vi "FGV_Calibration_KeyParams.vi"(7 "Action":T5, 8 "error in (no error)":errorcluster, 10 "GFG varname (Query)":string, 11 "System Type":string) -> (0 "error out":errorcluster, 1 "Imaging Reso Key Parameters":T4, 2 "Imaging Galvo Key Parameters":T4, 3 "Stimulating Galvo Key Parameters":T4, 4 "GFG Value requested":variant, 5 "Error Status Array (Empty on no error)":T1[](array[typedef]))   [LabVIEW 2012]
uses:
  Custom Controls and Typedefs/FGV_CalibrationKeyParams_Actions.ctl
  Custom Controls and Typedefs/Calibration Key Param structure.ctl
  <vilib>/Utility/VariantDataType/Type.ctl
  GFG/GFG Translator Wrapper/GFGTranslator_errors.ctl
  Custom Controls and Typedefs/Galvo Key Parameters.ctl
  Custom Controls and Typedefs/Reso Key Parameters.ctl
  Custom Controls and Typedefs/Galvo (Stim Path) Key Parameters.ctl
  GFG/GFG Translator Wrapper/GFGTranslator_Action.ctl
  GFG/GFG Translator Wrapper/GFGTranslator_Datatype.ctl
  Global_CalibrationSimulation.vi
  <vilib>/Utility/config.llb/Read Key (Double).vi
  <vilib>/Utility/config.llb/Read Key (Boolean).vi
  <vilib>/Utility/config.llb/NI_LVConfig.lvlib
  <vilib>/Utility/VariantDataType/VariantType.lvlib
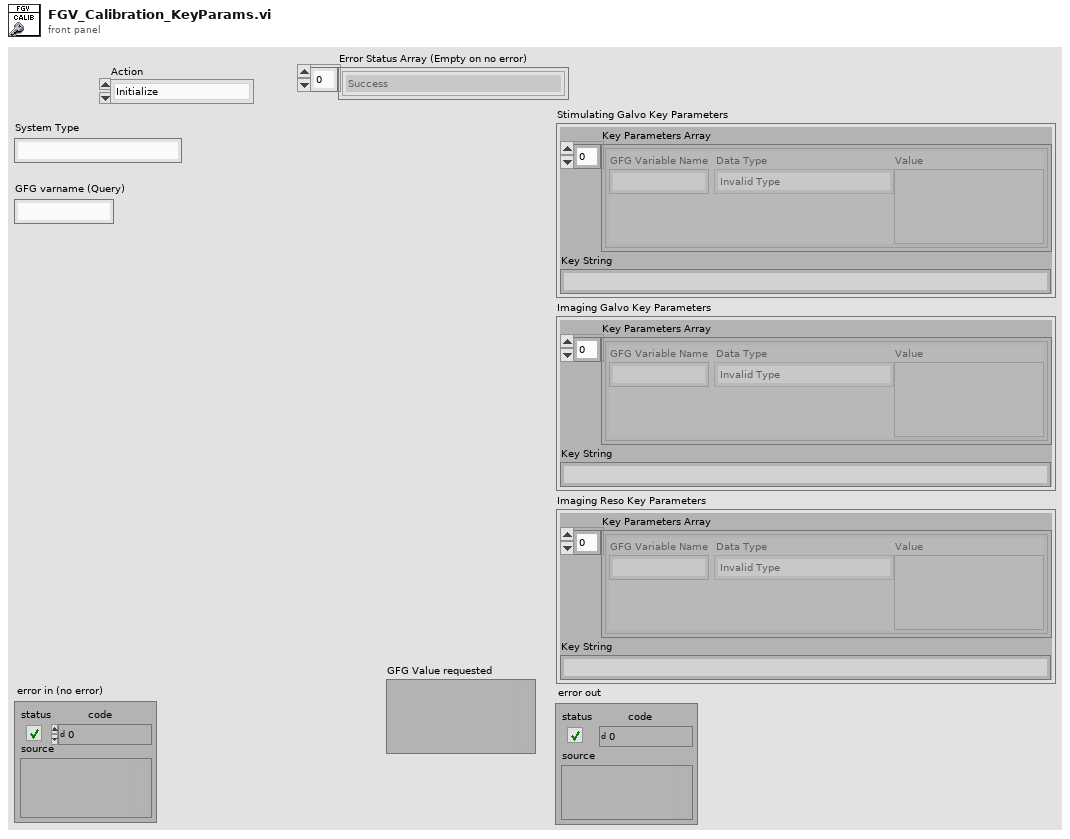
[diagram p1: front panel]
types:
  T1 = typedef "GFGTranslator_errors.ctl" = enum16{"Success", "SciScan Not Running", "No Get Method for Selected Datatype", "No Set Method for Selected Datatype", "Variable Not Found", "Unexpected Datatype", "Data Out of Range"}
  T2 = typedef "Calibration Key Param structure.ctl" = cluster{"GFG Variable Name":string, "Data Type":T3, "Value":variant}
  T3 = typedef "VariantType.lvlib/Type.ctl" = enum8{"Invalid Type", "Void", "I8", "I16", "I32", "I64", "U8", "U16", "U32", "U64", "Single Float", "Double Float", "Extended Float", "Single Complex", "Double Complex", "Extended Complex", "Enum U8", "Enum U16", "Enum U32", "Enum U64", "Single Float With Unit", "Double Float With Unit", "Extended Float With Unit", "Single Complex with Unit", "Double Complex with Unit", "Extended Complex with Unit", "Boolean", "String", "Path", "Picture", "Tag", "Array", "Cluster", "Variant", "LV Variant", "Waveform", "Timestamp", "Digital Waveform", "Digital Data", "ExpressData", "Refnum", "External Data", "VI", "Poly VI", "LabVIEW Class Instance", "Fixed Point"}
  T4 = cluster{"Key Parameters Array":T2[], "Key String":string}
  T5 = typedef "FGV_CalibrationKeyParams_Actions.ctl" = enum16{"Initialize", "Grab From SciScan and Store", "Read Parameters", "ReadGFGValue"}
  T6 = typedef "Galvo (Stim Path) Key Parameters.ctl" = T2[]
  T7 = typedef "Reso Key Parameters.ctl" = T2[]
  T8 = typedef "Galvo Key Parameters.ctl" = T2[]
  T9 = typedef "GFGTranslator_Datatype.ctl" = enum16{"String", "Path (String)", "Numeric", "Boolean", "Set_BoolRef (use boolean data)", "Get_Variant", "Get_2DArray (I16)", "Get_Image_2DArray (I16)", "Get_Version (String)", "Get_All GFG variables (String)"}
  T10 = typedef "GFGTranslator_Action.ctl" = enum16{"Get", "Set"}
  T11 = typedef "NI_LVConfig.lvlib/Config Data RefNum.ctl" = refnum<k1>
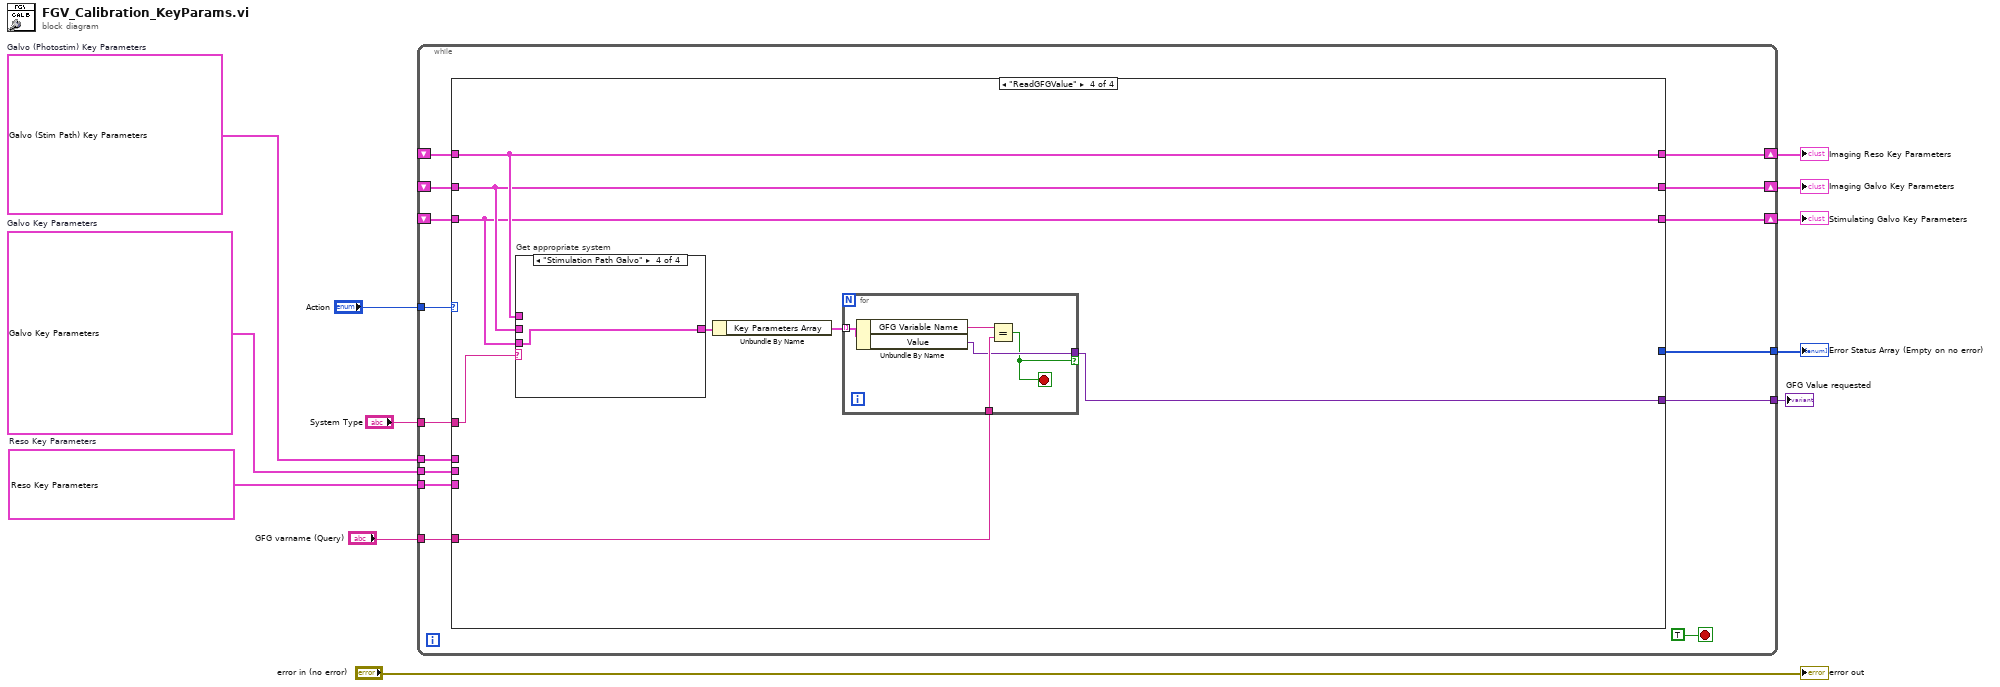
[diagram p0: block diagram]
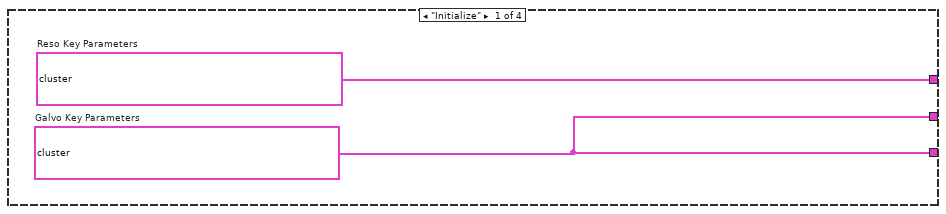
[diagram p2: hidden frame]
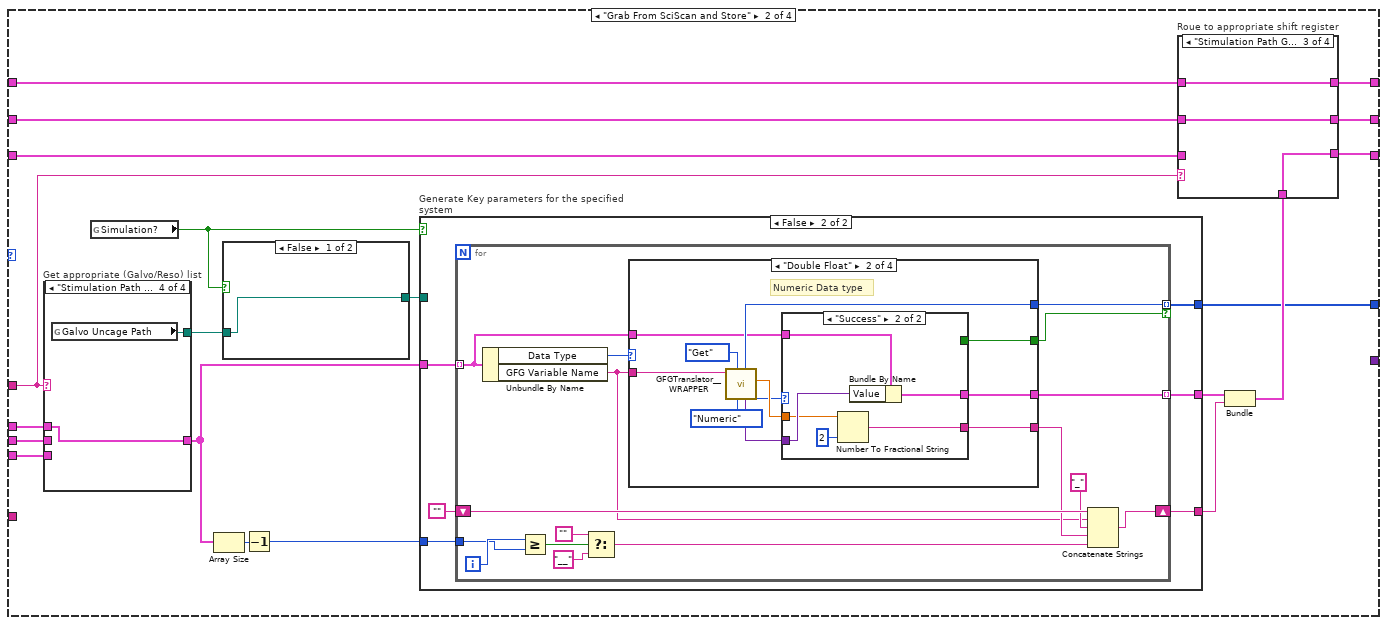
[diagram p3: hidden frame]
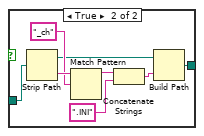
[diagram p4: hidden frame]
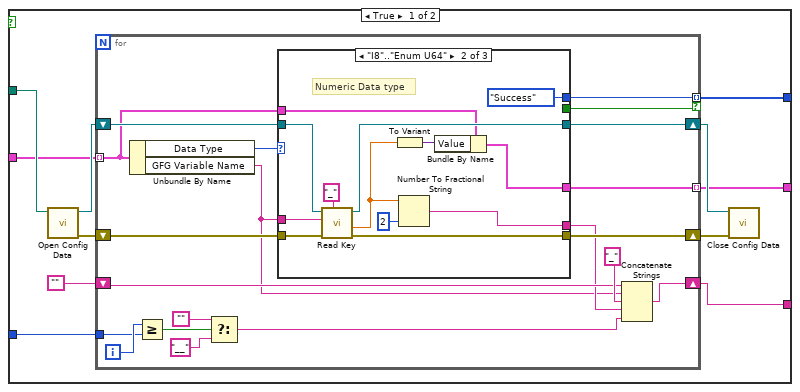
[diagram p5: hidden frame]
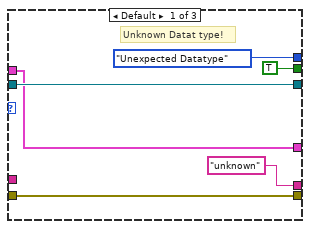
[diagram p6: hidden frame]
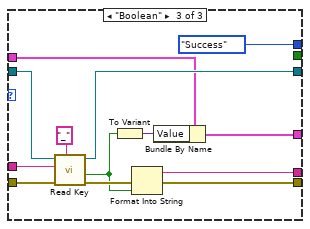
[diagram p7: hidden frame]
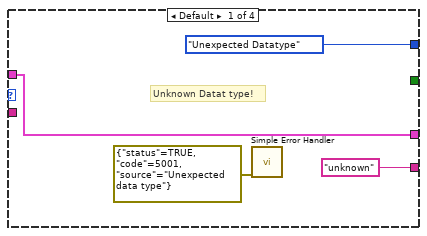
[diagram p8: hidden frame]
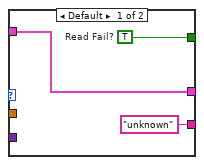
[diagram p9: hidden frame]
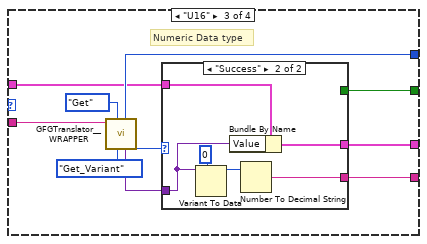
[diagram p10: hidden frame]
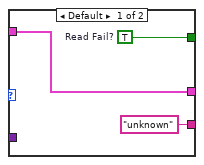
[diagram p11: hidden frame]
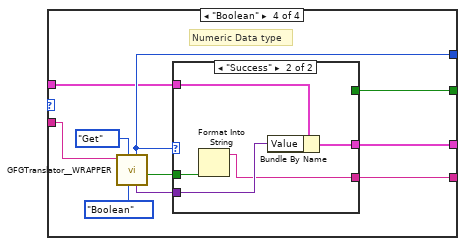
[diagram p12: hidden frame]
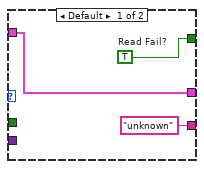
[diagram p13: hidden frame]
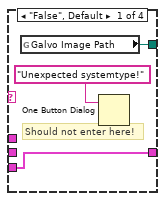
[diagram p14: hidden frame]
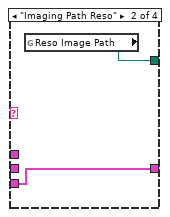
[diagram p15: hidden frame]
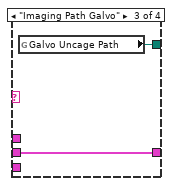
[diagram p16: hidden frame]
diagram:
  w3 = T6 [{"GFG Variable Name"="x.voltage", "Data Type"=enum."Double Float", "Value"=variant}, {"GFG Variable Name"="y.voltage", "Data Type"=enum."Double Float", "Value"=variant}, {"GFG Variable Name"="x.volt.offset", "Data Type"=enum."Double Float", "Value"=variant}, {"GFG Variable Name"="y.volt.offset", "Data Type"=enum."Double Float", "Value"=variant}, {"GFG Variable Name"="fill.fraction", "Data Type"=enum."Double Float", "Value"=variant}, {"GFG Variable Name"="x.invert.image", "Data Type"=enum."Boolean", "Value"=variant}, {"GFG Variable Name"="y.invert.image", "Data Type"=enum."Boolean", "Value"=variant}]  # Galvo (Photostim) Key Parameters
  w8 = T7 [{"GFG Variable Name"="x.voltage", "Data Type"=enum."Double Float", "Value"=variant}, {"GFG Variable Name"="y.voltage", "Data Type"=enum."Double Float", "Value"=variant}, {"GFG Variable Name"="x.correction", "Data Type"=enum."Double Float", "Value"=variant}]  # Reso Key Parameters
  w9 = T8 [{"GFG Variable Name"="x.voltage", "Data Type"=enum."Double Float", "Value"=variant}, {"GFG Variable Name"="y.voltage", "Data Type"=enum."Double Float", "Value"=variant}, {"GFG Variable Name"="x.volt.offset", "Data Type"=enum."Double Float", "Value"=variant}, {"GFG Variable Name"="y.volt.offset", "Data Type"=enum."Double Float", "Value"=variant}, {"GFG Variable Name"="speed.mode", "Data Type"=enum."U16", "Value"=variant}, {"GFG Variable Name"="fill.fraction", "Data Type"=enum."Double Float", "Value"=variant}, {"GFG Variable Name"="x.bidirectional", "Data Type"=enum."Boolean", "Value"=variant}, {"GFG Variable Name"="y.bidirectional", "Data Type"=enum."Boolean", "Value"=variant}, {"GFG Variable Name"="x.invert.image", "Data Type"=enum."Boolean", "Value"=variant}, {"GFG Variable Name"="y.invert.image", "Data Type"=enum."Boolean", "Value"=variant}]  # Galvo Key Parameters
  n1 = while {
    tunnel: "Action" -> [w26]
    tunnel: "System Type" -> [w22]
    shift-right: [w23] -> w5
    shift-left: _ -> [w21]
    shift-right: [w24] -> w6
    shift-left: _ -> [w20]
    shift-right: [w25] -> w7
    shift-left: _ -> [w19]
    tunnel: w9 -> [w18]
    tunnel: w8 -> [w17]
    tunnel: [w16] -> w4
    tunnel: w3 -> [w15]
    tunnel: "GFG varname (Query)" -> [w14]
    tunnel: [w13] -> w1
    stop <- TRUE stop-if-true
    n2 = case shown="\"ReadGFGValue\"" w26 {
      tunnel: [w28 w36 w224 w232] -> w25
      tunnel: [w28 w40 w225 w233] -> w24
      tunnel: [w29 w35 w226 w234] -> w23
      tunnel: w22 -> [_ w46 _ w231]
      tunnel: w21 -> [_ w49 w226 w234]
      tunnel: w20 -> [_ w48 w225 w233]
      tunnel: w19 -> [_ w47 w224 w232]
      tunnel: w18 -> [_ w43 _ _]
      tunnel: w17 -> [_ w42 _ _]
      tunnel: [_ w34 _ _] -> w16
      tunnel: w15 -> [_ w30 _ _]
      tunnel: w14 -> [_ _ _ w228]
      tunnel: [_ _ _ w227] -> w13
      frame "Initialize" {
        w29 = T4 {"Key Parameters Array"=[{"GFG Variable Name"="x.voltage", "Data Type"=enum."Double Float", "Value"=variant}, {"GFG Variable Name"="y.voltage", "Data Type"=enum."Double Float", "Value"=variant}, {"GFG Variable Name"="x.correction", "Data Type"=enum."Double Float", "Value"=variant}, {"GFG Variable Name"="Start.Delay", "Data Type"=enum."Double Float", "Value"=variant}], "Key String"="__"}  # Reso Key Parameters
        w28 = T4 {"Key Parameters Array"=[{"GFG Variable Name"="x.voltage", "Data Type"=enum."Double Float", "Value"=variant}, {"GFG Variable Name"="y.voltage", "Data Type"=enum."Double Float", "Value"=variant}, {"GFG Variable Name"="x.volt.offset", "Data Type"=enum."Double Float", "Value"=variant}, {"GFG Variable Name"="y.volt.offset", "Data Type"=enum."Double Float", "Value"=variant}, {"GFG Variable Name"="Start.Delay", "Data Type"=enum."Double Float", "Value"=variant}, {"GFG Variable Name"="speed.mode", "Data Type"=enum."U16", "Value"=variant}, {"GFG Variable Name"="fill.fraction", "Data Type"=enum."Double Float", "Value"=variant}, {"GFG Variable Name"="x.bidirectional", "Data Type"=enum."Boolean", "Value"=variant}, {"GFG Variable Name"="y.bidirectional", "Data Type"=enum."Boolean", "Value"=variant}], "Key String"="__"}  # Galvo Key Parameters
      }
      frame "Grab From SciScan and Store" {
        n3 = case "Get appropriate (Galvo/Reso) list" shown="\"Stimulation Path Galvo\"" w46 {
          tunnel: w43 -> [_ _ w209 _]
          tunnel: w42 -> [w204 w207 _ _]
          tunnel: [w204 w207 w209 w210] -> w41
          tunnel: [w203 w206 w208 w211] -> w32
          tunnel: w30 -> [_ _ _ w210]
          frame "False", Default {
            # "Should not enter here!"
            n4 = global read "Global_CalibrationSimulation.vi" "Galvo Image Path"() -> (w203:path)
            n5 = One Button Dialog(message="Unexpected systemtype!") -> ()  [unwired: 1 in, 1 out]
          }
          frame "Imaging Path Reso" {
            n6 = global read "Global_CalibrationSimulation.vi" "Reso Image Path"() -> (w206:path)
          }
          frame "Imaging Path Galvo" {
            n7 = global read "Global_CalibrationSimulation.vi" "Galvo Uncage Path"() -> (w208:path)
          }
          frame "Stimulation Path Galvo" {
            n8 = global read "Global_CalibrationSimulation.vi" "Galvo Uncage Path"() -> (w211:path)
          }
        }
        n9 = global read "Global_CalibrationSimulation.vi" "Simulation?"() -> (w33:bool)
        n10 = Array Size(array=w41) -> (size(s)=w45:i32)
        n11 = case shown="False" w33 {
          tunnel: w32 -> [w50 w52]
          tunnel: [w50 w51] -> w31
          frame False {
          }
          frame True {
            n12 = Strip Path(path=w52) -> (stripped path=w54:path, name=w57:string)
            n13 = Match Pattern(string=w57, regular expression="_ch" ("search string")) -> (before substring=w55:string)  [unwired: 1 in, 3 out]
            n14 = Concatenate Strings(w55, ".INI" ("string")) -> (w53:string)
            n15 = Build Path(base path=w54, name or relative path=w53) -> (appended path=w51:path)
          }
        }
        n16 = Decrement(x=w45) -> (x-1=w44:i32)
        n17 = case "Generate Key parameters for the specified system" shown="False" w33 {
          tunnel: w31 -> [w69 _]
          tunnel: [w64 w127] -> w34
          tunnel: [w59 w126] -> w39
          tunnel: w44 -> [w62 w124]
          tunnel: [w60 w123] -> w38
          tunnel: w41 -> [w63 w122]
          frame True {
            n18 = call <vilib>:"Open Config Data.vi"("configuration file path"=w69) -> ("error out"=w67:errorcluster, "refnum"=w68:T11)  [unwired: 8 in, 1 out]
            n19 = for {
              shift-right: [w88] -> w65
              shift-left: w68 -> [w89]
              shift-right: [w86] -> w66
              shift-left: w67 -> [w87]
              tunnel: [w85] -> w64 mode=indexing if=w84
              tunnel: w63 -> [w73] mode=indexing
              tunnel: w62 -> [w80]
              shift-right: [w74] -> w60
              shift-left: "" -> [w78]
              tunnel: [w72] -> w59 mode=indexing
              i -> [w81]
              n20 = Unbundle By Name(w73) -> ("Data Type"=w83:T3, "GFG Variable Name"=w76:string)
              n21 = Greater Or Equal?(x=w81, y=w80) -> (x >= y?=w82:bool)
              n22 = Select(t="", s=w82, f="__" ("t")) -> (s? t:f=w75:string)
              n23 = case shown="\"I8\"..\"Enum U64\"" w83 {
                tunnel: w76 -> [_ w102 w116]
                tunnel: w89 -> [w94 w107 w120]
                tunnel: [w94 w106 w119] -> w88
                tunnel: w87 -> [w95 w105 w118]
                tunnel: [w95 w103 w113] -> w86
                tunnel: [GFGTranslator_errors."Unexpected Datatype" ("Status Output") GFGTranslator_errors."Success" ("Status Output") GFGTranslator_errors."Success" ("Status Output")] -> w85
                tunnel: [TRUE _ _] -> w84
                tunnel: ["unknown" w100 w114] -> w77
                tunnel: w73 -> [w91 w99 w112]
                tunnel: [w91 w96 w109] -> w72
                frame Default {
                  # "Unknown Datat type!"
                }
                frame "I8".."Enum U64" {
                  # "Numeric Data type"
                  n24 = call-poly <vilib>:"Read Key.vi"("section"="_", "error in (no error)"=w105, "key"=w102, "refnum"=w107) -> ("error out"=w103:errorcluster, "value"=w97:dbl, "refnum out"=w106:T11)  [unwired: 4 in, 1 out]
                  n25 = To Variant(anything=w97) -> (Variant=w98:variant)
                  n26 = Number To Fractional String(number=w97, precision (6)=i16 2) -> (F-format string=w100:string)  [unwired: 2 in]
                  n27 = Bundle By Name(cluster=w99, "Value"=w98) -> (w96:T2)
                }
                frame "Boolean" {
                  n28 = call-poly <vilib>:"Read Key.vi"("section"="_", "error in (no error)"=w118, "key"=w116, "refnum"=w120) -> ("error out"=w115:errorcluster, "value"=w111:bool, "refnum out"=w119:T11)  [unwired: 4 in, 1 out]
                  n29 = To Variant(anything=w111) -> (Variant=w110:variant)
                  n30 = Format Into String(error in=w115, w111) -> (resulting string=w114:string, error out=w113:errorcluster)  [unwired: 2 in]
                  n31 = Bundle By Name(cluster=w112, "Value"=w110) -> (w109:T2)
                }
              }
              n32 = Concatenate Strings(w78, w76, "_" ("string"), w77, w75) -> (w74:string)
            }
            n33 = call <vilib>:"Close Config Data.vi"("error in (no error)"=w66, "refnum"=w65) -> ()  [unwired: 8 in, 2 out]
          }
          frame False {
            n34 = for {
              tunnel: [w143] -> w127 mode=indexing if=w142
              tunnel: [w141] -> w126 mode=indexing
              shift-right: [w134] -> w123
              shift-left: "" -> [w140]
              tunnel: w124 -> [w137]
              tunnel: w122 -> [w132] mode=indexing
              i -> [w138]
              n35 = Unbundle By Name(w132) -> ("Data Type"=w133:T3, "GFG Variable Name"=w130:string)
              n36 = Greater Or Equal?(x=w138, y=w137) -> (x >= y?=w136:bool)
              n37 = Select(t="", s=w136, f="__" ("t")) -> (s? t:f=w135:string)
              n38 = case shown="\"Double Float\"" w133 {
                tunnel: w130 -> [_ w148 w167 w185]
                tunnel: [GFGTranslator_errors."Unexpected Datatype" ("Status Output") w154 w173 w192] -> w143
                tunnel: [_ w153 w172 w191] -> w142
                tunnel: [w144 w151 w170 w187] -> w141
                tunnel: ["unknown" w150 w169 w186] -> w139
                tunnel: w132 -> [w144 w149 w168 w189]
                frame Default {
                  # "Unknown Datat type!"
                  n39 = call <vilib>:"Simple Error Handler.vi"("error in (no error)"=errorcluster {"status"=TRUE, "code"=5001, "source"="Unexpected data type"} ("error constant")) -> ()  [unwired: 4 in, 5 out]
                }
                frame "Double Float" {
                  # "Numeric Data type"
                  n40 = call "GFGTranslator__WRAPPER.vi"("GFGTranslator Datatype"=GFGTranslator_Datatype."Numeric", "GFG Translator Action"=GFGTranslator_Action."Get", "GFG Variable Name"=w148) -> ("Numeric_Output"=w155:dbl, "Variant_Output"=w152:variant, "Status Output"=w154:T1)  [unwired: 3 in, 3 out]
                  n41 = case shown="\"Success\"" w154 {
                    tunnel: w155 -> [_ w164]
                    tunnel: [w160 _] -> w153
                    tunnel: w152 -> [_ w166]
                    tunnel: [w159 w165] -> w151
                    tunnel: ["unknown" w162] -> w150
                    tunnel: w149 -> [w159 w161]
                    frame Default {
                      w160 = TRUE  # Read Fail?
                    }
                    frame "Success" {
                      n42 = Number To Fractional String(number=w164, precision (6)=i16 2) -> (F-format string=w162:string)  [unwired: 2 in]
                      n43 = Bundle By Name(cluster=w161, "Value"=w166) -> (w165:T2)
                    }
                  }
                }
                frame "U16" {
                  # "Numeric Data type"
                  n44 = call "GFGTranslator__WRAPPER.vi"("GFGTranslator Datatype"=GFGTranslator_Datatype."Get_Variant", "GFG Translator Action"=GFGTranslator_Action."Get", "GFG Variable Name"=w167) -> ("Variant_Output"=w171:variant, "Status Output"=w173:T1)  [unwired: 3 in, 4 out]
                  n45 = case shown="\"Success\"" w173 {
                    tunnel: [w178 _] -> w172
                    tunnel: w171 -> [_ w181]
                    tunnel: [w177 w184] -> w170
                    tunnel: ["unknown" w183] -> w169
                    tunnel: w168 -> [w177 w182]
                    frame Default {
                      w178 = TRUE  # Read Fail?
                    }
                    frame "Success" {
                      n46 = Variant To Data(type=u16 0 ("number"), Variant=w181) -> (data=w179:u16)  [unwired: 1 in, 1 out]
                      n47 = Bundle By Name(cluster=w182, "Value"=w181) -> (w184:T2)
                      n48 = Number To Decimal String(number=w179) -> (decimal integer string=w183:string)  [unwired: 1 in]
                    }
                  }
                }
                frame "Boolean" {
                  # "Numeric Data type"
                  n49 = call "GFGTranslator__WRAPPER.vi"("GFGTranslator Datatype"=GFGTranslator_Datatype."Boolean", "GFG Translator Action"=GFGTranslator_Action."Get", "GFG Variable Name"=w185) -> ("Boolean_Output"=w190:bool, "Variant_Output"=w188:variant, "Status Output"=w192:T1)  [unwired: 3 in, 3 out]
                  n50 = case shown="\"Success\"" w192 {
                    tunnel: [w197 _] -> w191
                    tunnel: w190 -> [_ w200]
                    tunnel: w189 -> [w195 w202]
                    tunnel: w188 -> [_ w201]
                    tunnel: [w195 w199] -> w187
                    tunnel: ["unknown" w198] -> w186
                    frame Default {
                      w197 = TRUE  # Read Fail?
                    }
                    frame "Success" {
                      n51 = Format Into String(w200) -> (resulting string=w198:string)  [unwired: 3 in, 1 out]
                      n52 = Bundle By Name(cluster=w202, "Value"=w201) -> (w199:T2)
                    }
                  }
                }
              }
              n53 = Concatenate Strings(w140, w130, "_" ("string"), w139, w135) -> (w134:string)
            }
          }
        }
        n54 = Bundle(w39, w38) -> (w37:cluster{T2[], string})  [unwired: 1 in]
        n55 = case "Roue to appropriate shift register" shown="\"Stimulation Path Galvo\"" w46 {
          tunnel: w49 -> [w214 w215 w218 _]
          tunnel: w48 -> [w213 _ w219 w222]
          tunnel: w47 -> [w212 w216 _ w221]
          tunnel: w37 -> [_ w217 w220 w223]
          tunnel: [w213 w217 w219 w222] -> w40
          tunnel: [w212 w216 w220 w221] -> w36
          tunnel: [w214 w215 w218 w223] -> w35
          frame "False", Default {
          }
          frame "Imaging Path Galvo" {
          }
          frame "Stimulation Path Galvo" {
          }
          frame "Imaging Path Reso" {
          }
        }
      }
      frame "Read Parameters", Default {
      }
      frame "ReadGFGValue" {
        n56 = case "Get appropriate system" shown="\"Stimulation Path Galvo\"" w231 {
          tunnel: [T4 {"Key Parameters Array"=[], "Key String"=""} ("Galvo Key Parameters") w242 w243 w244] -> w230
          tunnel: w234 -> [_ w242 _ _]
          tunnel: w233 -> [_ _ w243 _]
          tunnel: w232 -> [_ _ _ w244]
          frame "False", Default {
            # "Should not enter here!"
            n57 = One Button Dialog(message="Unexpected systemtype!") -> ()  [unwired: 1 in, 1 out]
          }
          frame "Imaging Path Reso" {
          }
          frame "Imaging Path Galvo" {
          }
          frame "Stimulation Path Galvo" {
          }
        }
        n58 = Unbundle By Name(w230) -> ("Key Parameters Array"=w229:T2[])
        n59 = for {
          tunnel: w229 -> [w239] mode=indexing
          tunnel: w228 -> [w237]
          tunnel: [w236] -> w227 if=w235
          stop <- w235 stop-if-true
          n60 = Unbundle By Name(w239) -> ("GFG Variable Name"=w238:string, "Value"=w236:variant)
          n61 = Equal?(x=w238, y=w237) -> (x = y?=w235:bool)
        }
      }
    }
  }
  "Stimulating Galvo Key Parameters" <- w7
  "Imaging Galvo Key Parameters" <- w6
  "Imaging Reso Key Parameters" <- w5
  "Error Status Array (Empty on no error)" <- w4
  "GFG Value requested" <- w1
  "error out" <- "error in (no error)"
